vi "Start BuildWorker.vi"(8 "error in (no error)":errorcluster, 9 "Show":bool=TRUE, 10 "Port":i32=4545, 11 "BuildWorker in":refnum<class "BuildWorker.lvclass">) -> (0 "error out":errorcluster, 3 "BuildWorker out":refnum<class "BuildWorker.lvclass">)   [LabVIEW 2017, in "BuildWorker Interface.lvlib" / "BuildWorker.lvclass"]
uses:
  BuildWorker.lvclass
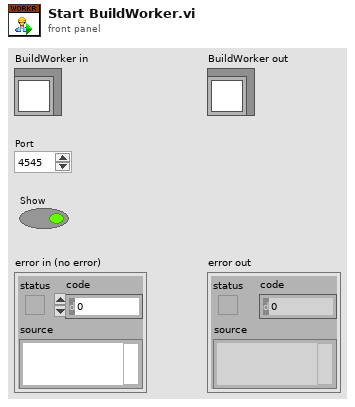
[diagram p1: front panel]
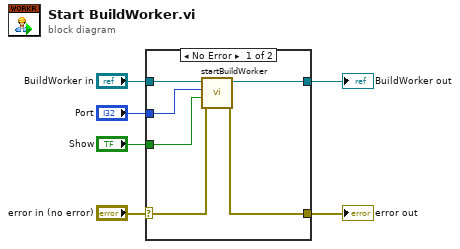
[diagram p0: block diagram]
diagram:
  n1 = case shown="No Error" "error in (no error)" {
    selector: "error in (no error)" -> [w10 w14]
    tunnel: "BuildWorker in" -> [w12 w13]
    tunnel: [w11 w13] -> w5
    tunnel: [w9 w14] -> w3
    tunnel: "Port" -> [w8 _]
    tunnel: "Show" -> [w7 _]
    frame No Error {
      n2 = call-dynamic "startBuildWorker.vi"("error in (no error)"=w10, "Show"=w7, "Port"=w8, "BuildWorker in"=w12) -> ("error out"=w9:errorcluster, "BuildWorker out"=w11:refnum<class "BuildWorker.lvclass">)  [unwired: 6 in]
    }
    frame Error {
    }
  }
  "error out" <- w3
  "BuildWorker out" <- w5
